vi "PumpValveHeater.vi"() -> ()   [LabVIEW 2015]
uses:
  PumpValve.ctl
  <vilib>/DAQmx/write.llb/DAQmx Write (Digital 1D Bool NChan 1Samp 1Line).vi
  <vilib>/DAQmx/miscellaneous.llb/DAQmx Fill In Error Info.vi
panel:
  in  "On/Off Temp":bool
  in  "Manual Mode Temp":bool
  in  "stop controller":bool
  in  "Set Temp":bool
  in  "Duty cycle % (0-100)":dbl=50.0
  in  "stop PWM":bool
  in  "Steps in a cycle":i32=256
  in  "Cycle time (s)":i32=5
  in  "On/Off (Pump)":bool
  in  "Open/Close (Blue)":bool
  in  "Open/Close (Green)":bool
  in  "Manual Mode Pump/Valve":bool
  out "Invalid fill%":bool
  out "Tank":u32(slide) scale=0.0..100.0
  in  "Drain %":u32
  in  "Fill %":u32
  in  "Drain":bool
  in  "Stop Program":bool
  in  "Fill":bool
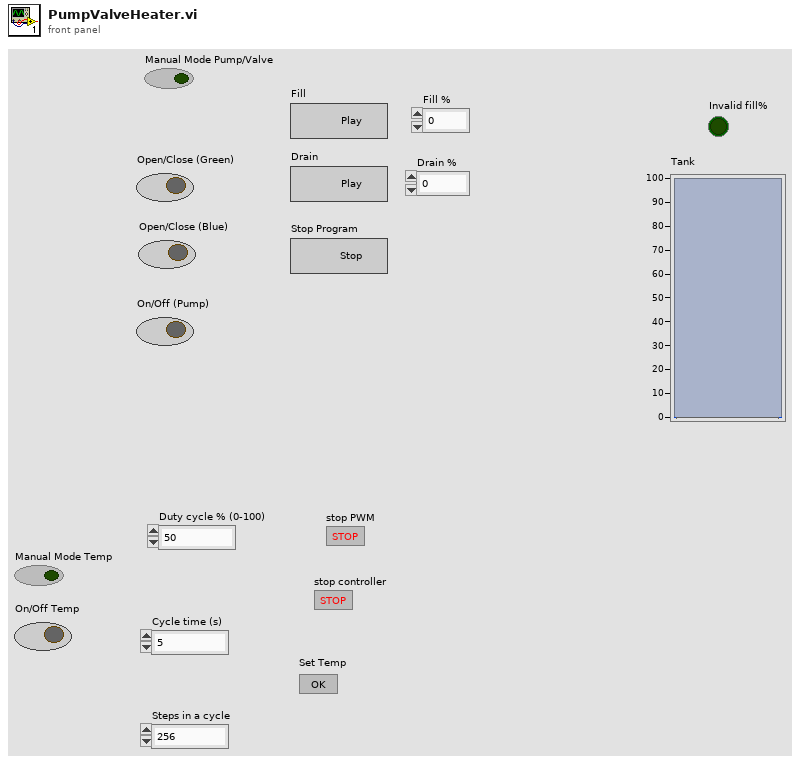
[diagram p1: front panel]
types:
  T1 = typedef "PumpValve.ctl" = enum16{"ManualTemp", "Idle Temp", "Set Temp", "Initialize", "Idle", "Fill", "Drain", "Stop"}
  T2 = cluster{"Open/Close (Green)":bool, "Open/Close (Blue)":bool, "On/Off (Pump)":bool}
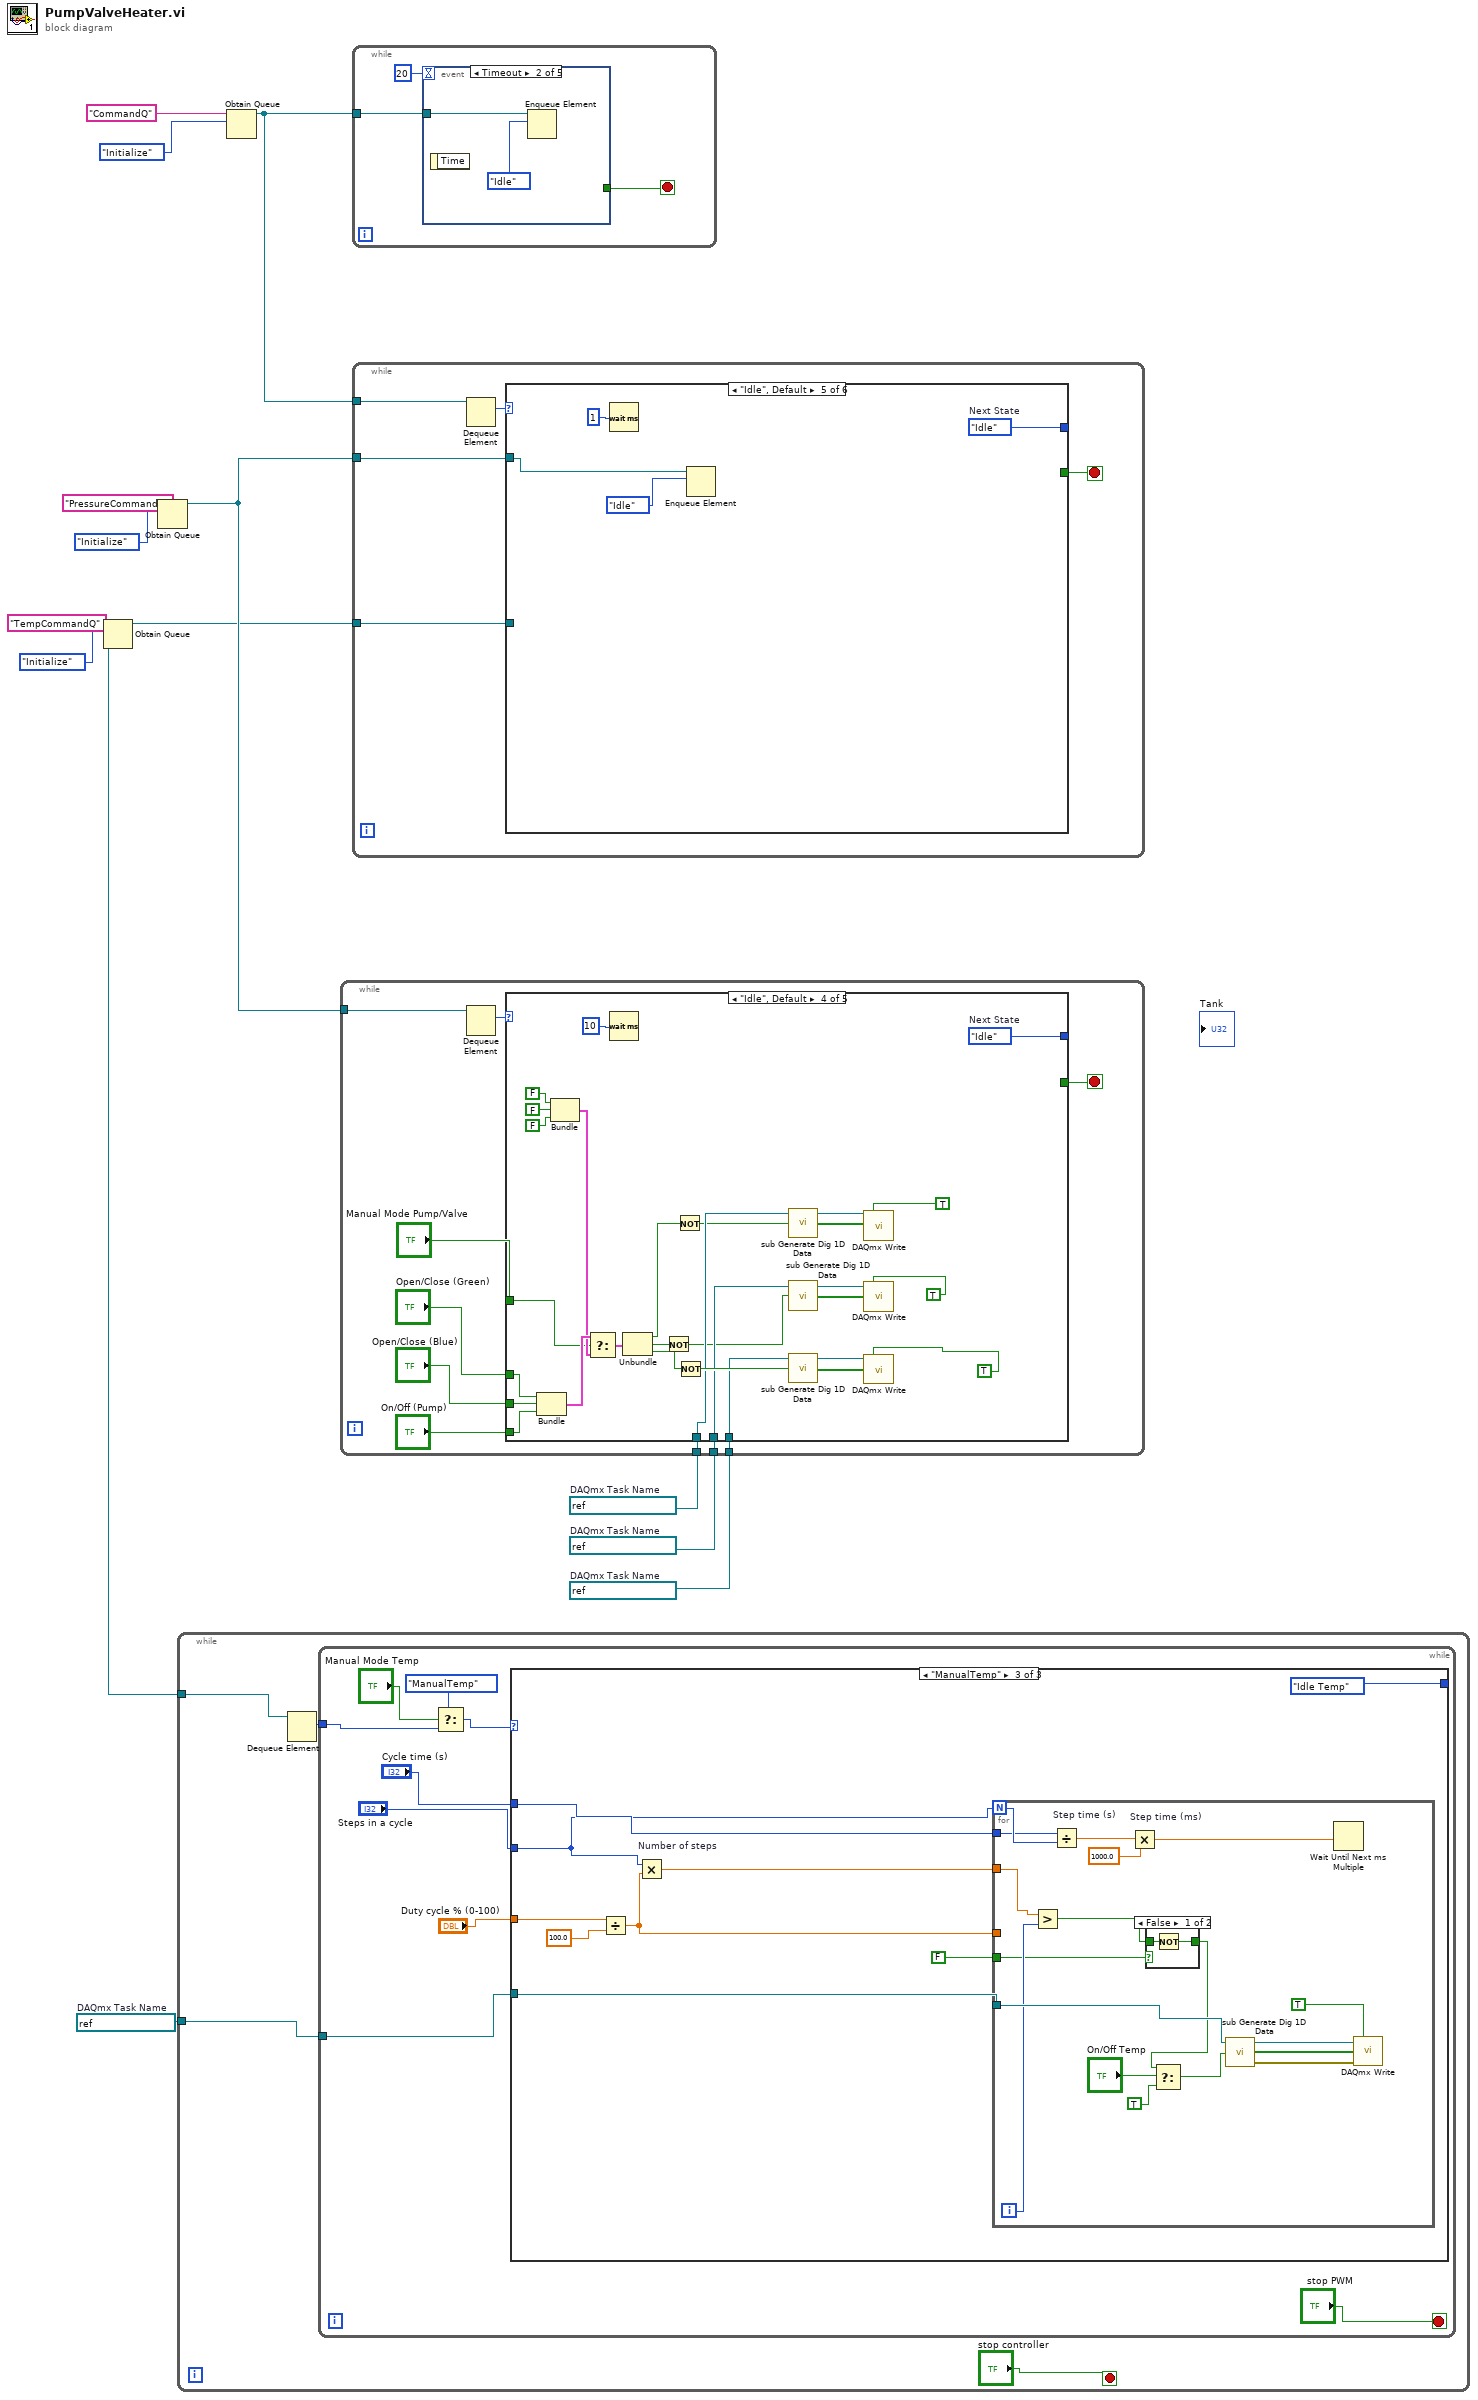
[diagram p0: block diagram]
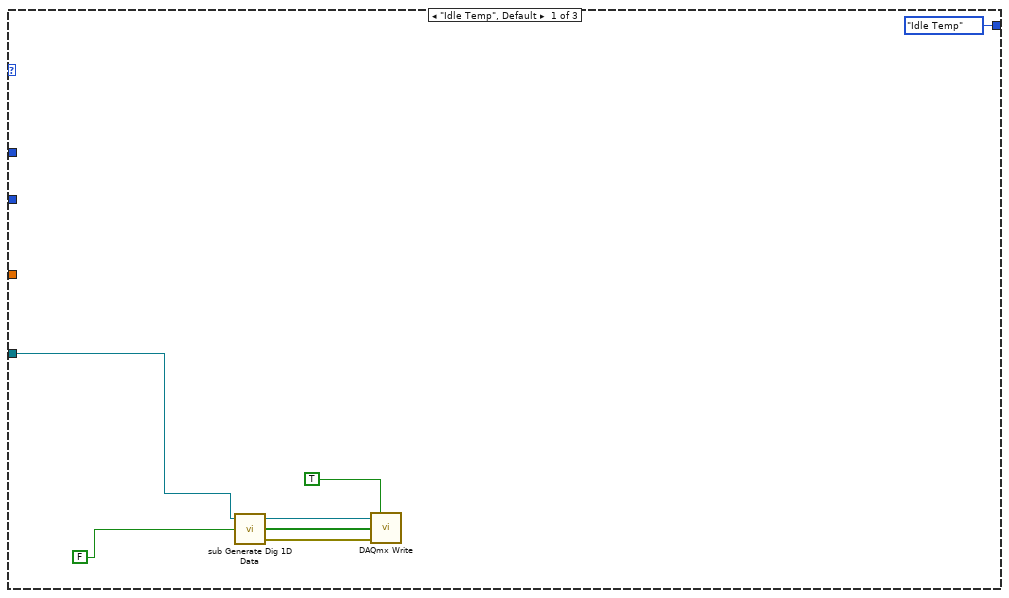
[diagram p2: hidden frame]
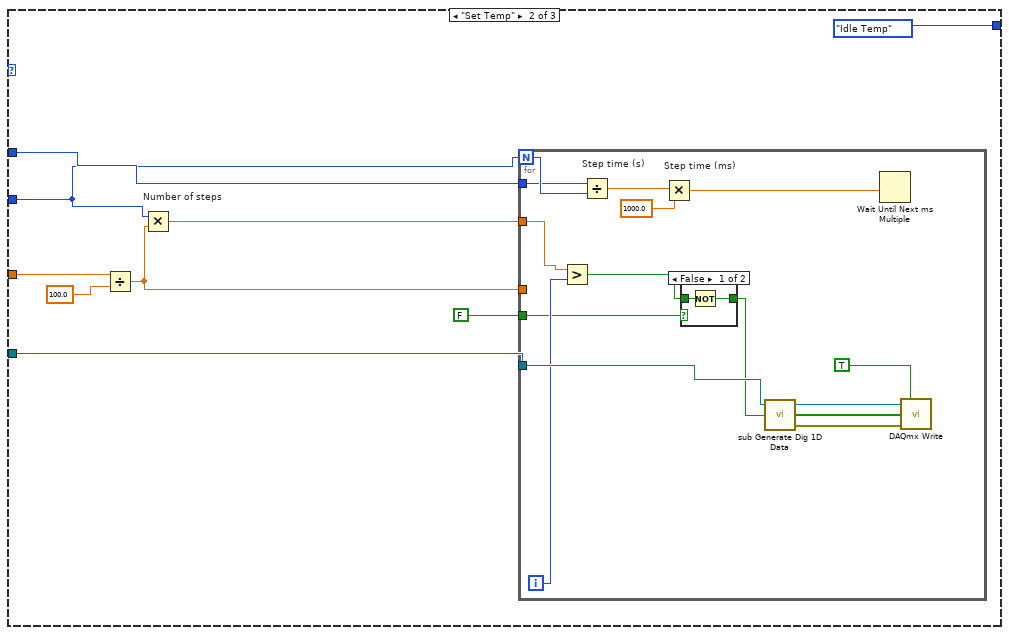
[diagram p3: hidden frame]
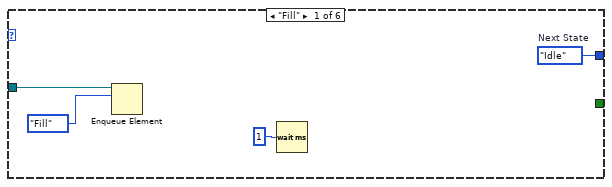
[diagram p6: hidden frame]
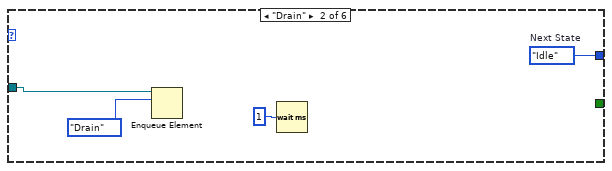
[diagram p7: hidden frame]
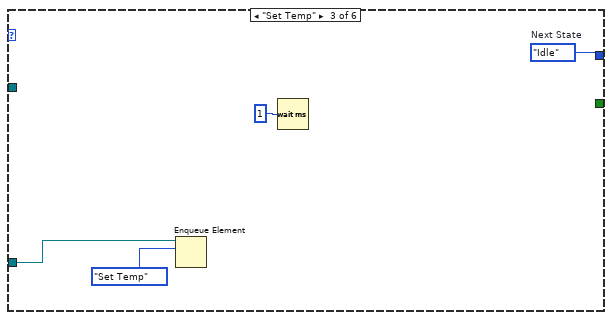
[diagram p8: hidden frame]
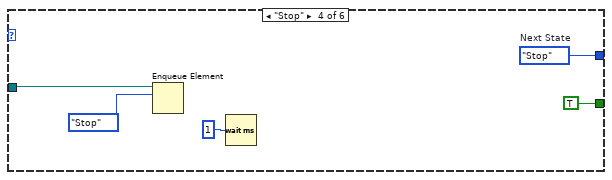
[diagram p9: hidden frame]
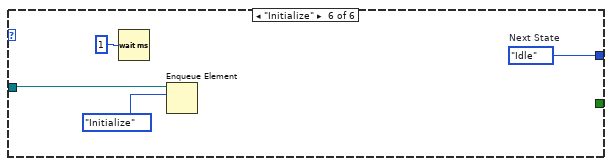
[diagram p10: hidden frame]
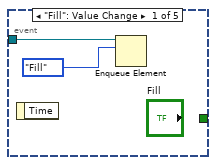
[diagram p11: hidden frame]
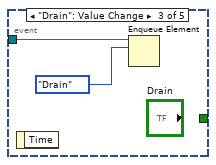
[diagram p12: hidden frame]
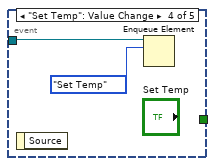
[diagram p13: hidden frame]
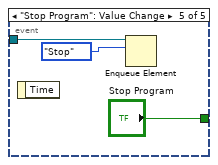
[diagram p14: hidden frame]
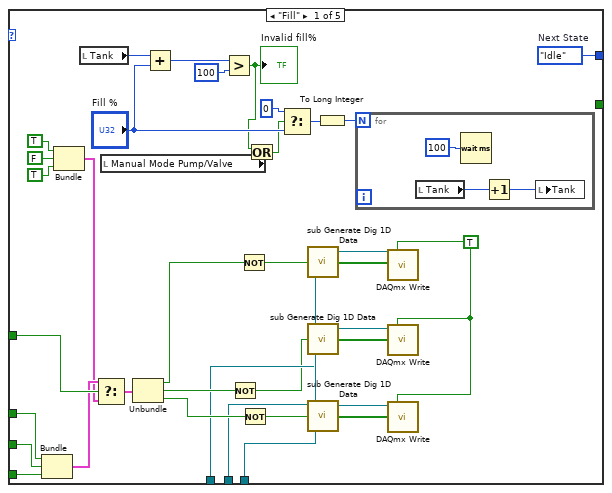
[diagram p15: hidden frame]
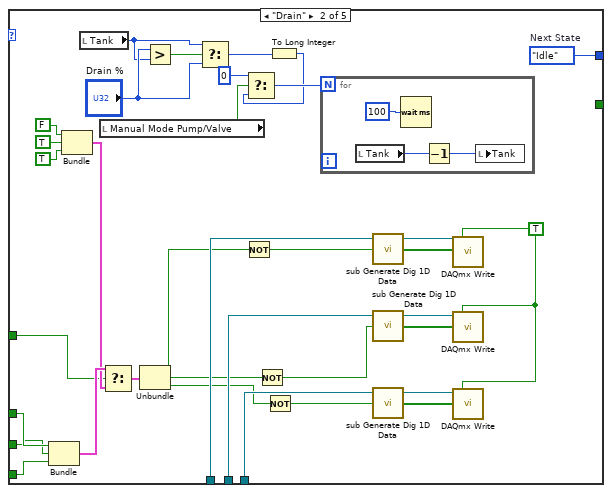
[diagram p16: hidden frame]
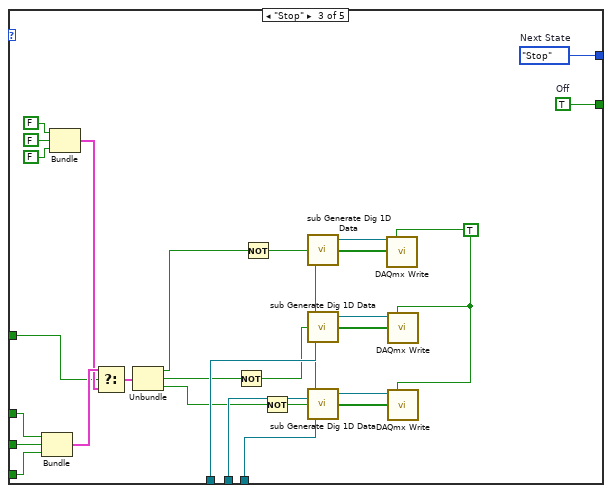
[diagram p17: hidden frame]
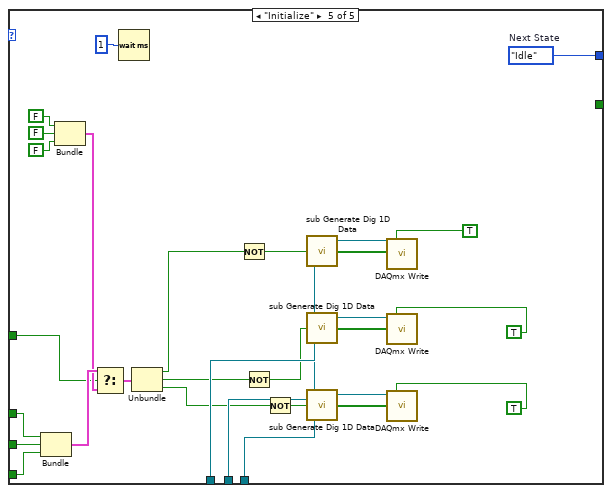
[diagram p18: hidden frame]
diagram:
  w4 = refnum<k21> "DigitalOutBlue"  # DAQmx Task Name
  w9 = refnum<k21> "DigitalOutGreen"  # DAQmx Task Name
  w10 = refnum<k21> "DigitalOutGreen"  # DAQmx Task Name
  w11 = refnum<k21> "DigitalOutGreen"  # DAQmx Task Name
  n1 = Obtain Queue(name (unnamed)="TempCommandQ", element data type=PumpValve."Initialize" ("States")) -> (queue out=w1:refnum<queue>)  [unwired: 3 in, 2 out]
  n2 = Obtain Queue(name (unnamed)="PressureCommandQ", element data type=PumpValve."Initialize" ("States")) -> (queue out=w5:refnum<queue>)  [unwired: 3 in, 2 out]
  n3 = while {
    tunnel: w4 -> [w17]
    tunnel: w1 -> [w16]
    stop <- "stop controller" stop-if-true
    n4 = Dequeue Element(queue=w16) -> (element=w15:T1)  [unwired: 2 in, 3 out]
    n5 = while {
      tunnel: w17 -> [w26]
      tunnel: w15 -> [w21]
      stop <- "stop PWM" stop-if-true
      n6 = Select(t=PumpValve."ManualTemp", s="Manual Mode Temp", f=w21) -> (s? t:f=w20:T1)
      n7 = case shown="\"ManualTemp\"" w20 {
        tunnel: w26 -> [w28 w42 w69]
        tunnel: [PumpValve."Idle Temp" ("States") PumpValve."Idle Temp" ("States") PumpValve."Idle Temp" ("States")] -> _
        tunnel: "Cycle time (s)" -> [_ w36 w63]
        tunnel: "Steps in a cycle" -> [_ w35 w62]
        tunnel: "Duty cycle % (0-100)" -> [_ w34 w61]
        frame "Idle Temp", Default {
          n8 = call <vilib>:"sub Generate Dig 1D Data.vi"("initial value"=FALSE, "task in"=w28) -> ("error out"=w30:errorcluster, "Data"=w31:bool[], "task out"=w32:refnum<k21>)  [unwired: 1 in]
          n9 = call-poly <vilib>:"DAQmx Write.vi"("task/channels in"=w32, "auto start"=TRUE, "data"=w31, "error in"=w30) -> ()  [unwired: 9 in, 3 out]
        }
        frame "Set Temp" {
          n10 = Divide(x=w34, y=100.0) -> (x/y=w40:dbl)
          n11 = Multiply "Number of steps"(x=w35, y=w40) -> (x*y=w39:dbl)
          n12 = for {
            N: w35 -> [w51]
            tunnel: w42 -> [w53]
            tunnel: w40 -> [_]
            tunnel: w36 -> [w50]
            tunnel: w39 -> [w46]
            tunnel: FALSE -> [w43]
            i -> [w45]
            n13 = Greater?(x=w46, y=w45) -> (0:w44:bool)
            n14 = Divide "Step time (s)"(x=w50, y=w51) -> (x/y=w49:dbl)
            n15 = Multiply "Step time (ms)"(x=w49, y=1000.0) -> (x*y=w47:dbl)
            n16 = case shown="False" w43 {
              tunnel: [w58 w60] -> w52
              tunnel: w44 -> [w59 w60]
              frame False {
                n17 = Not(x=w59) -> (.not. x?=w58:bool)
              }
              frame True {
              }
            }
            n18 = call <vilib>:"sub Generate Dig 1D Data.vi"("initial value"=w52, "task in"=w53) -> ("error out"=w56:errorcluster, "Data"=w55:bool[], "task out"=w54:refnum<k21>)  [unwired: 1 in]
            n19 = Wait Until Next ms Multiple(millisecond multiple=w47) -> ()  [unwired: 1 out]
            n20 = call-poly <vilib>:"DAQmx Write.vi"("task/channels in"=w54, "auto start"=TRUE, "data"=w55, "error in"=w56) -> ()  [unwired: 9 in, 3 out]
          }
        }
        frame "ManualTemp" {
          n21 = Divide(x=w61, y=100.0) -> (x/y=w67:dbl)
          n22 = Multiply "Number of steps"(x=w62, y=w67) -> (x*y=w66:dbl)
          n23 = for {
            N: w62 -> [w82]
            tunnel: w69 -> [w83]
            tunnel: w67 -> [_]
            tunnel: w63 -> [w81]
            tunnel: w66 -> [w77]
            tunnel: FALSE -> [w74]
            i -> [w76]
            n24 = Greater?(x=w77, y=w76) -> (0:w75:bool)
            n25 = Divide "Step time (s)"(x=w81, y=w82) -> (x/y=w80:dbl)
            n26 = Multiply "Step time (ms)"(x=w80, y=1000.0) -> (x*y=w78:dbl)
            n27 = case shown="False" w74 {
              tunnel: [w88 w90] -> w72
              tunnel: w75 -> [w89 w90]
              frame False {
                n28 = Not(x=w89) -> (.not. x?=w88:bool)
              }
              frame True {
              }
            }
            n29 = Select(t=w72, s="On/Off Temp", f=TRUE) -> (s? t:f=w71:bool)
            n30 = call <vilib>:"sub Generate Dig 1D Data.vi"("initial value"=w71, "task in"=w83) -> ("error out"=w86:errorcluster, "Data"=w85:bool[], "task out"=w84:refnum<k21>)  [unwired: 1 in]
            n31 = Wait Until Next ms Multiple(millisecond multiple=w78) -> ()  [unwired: 1 out]
            n32 = call-poly <vilib>:"DAQmx Write.vi"("task/channels in"=w84, "auto start"=TRUE, "data"=w85, "error in"=w86) -> ()  [unwired: 9 in, 3 out]
          }
        }
      }
    }
  }
  n33 = Obtain Queue(name (unnamed)="CommandQ", element data type=PumpValve."Initialize" ("States")) -> (queue out=w8:refnum<queue>)  [unwired: 3 in, 2 out]
  n34 = while {
    tunnel: w5 -> [w100]
    tunnel: w11 -> [w91]
    tunnel: w10 -> [w92]
    tunnel: w9 -> [w93]
    stop <- w99 stop-if-true
    n35 = Dequeue Element(queue=w100) -> (element=w98:T1)  [unwired: 2 in, 3 out]
    n36 = case shown="\"Idle\", Default" w98 {
      tunnel: [w137 w175 w206 w236 w266] -> _
      tunnel: [_ _ w179 _ _] -> w99
      tunnel: "Open/Close (Blue)" -> [w123 w151 w187 w219 w246]
      tunnel: "Open/Close (Green)" -> [w122 w152 w188 w220 w247]
      tunnel: "On/Off (Pump)" -> [w121 w150 w186 w218 w245]
      tunnel: "Manual Mode Pump/Valve" -> [w120 w153 w189 w221 w248]
      tunnel: w93 -> [w106 w147 w191 w211 w250]
      tunnel: w92 -> [w105 w148 w192 w210 w251]
      tunnel: w91 -> [w104 w149 w193 w209 w252]
      frame "Fill" {
        w116 = TRUE
        w137 = PumpValve."Idle"  # Next State
        n37 = Bundle("Open/Close (Green)"=w122, "Open/Close (Blue)"=w123, "On/Off (Pump)"=w121) -> (w119:T2)  [unwired: 1 in]
        n38 = Bundle(TRUE, FALSE, TRUE) -> (w118:cluster{bool, bool, bool})  [unwired: 1 in]
        n39 = local read "Tank"() -> (w136:u32)
        n40 = Select(t=w119, s=w120, f=w118) -> (s? t:f=w117:T2)
        n41 = local read "Manual Mode Pump/Valve"() -> (w125:bool)
        n42 = Unbundle(w117) -> ("Open/Close (Green)"=w109:bool, "Open/Close (Blue)"=w108:bool, "On/Off (Pump)"=w107:bool)
        n43 = Add(x=w136, y="Fill %") -> (x+y=w134:u32)
        n44 = Greater?(x=w134, y=u32 100) -> (0:w126:bool)
        "Invalid fill%" <- w126
        n45 = Not(x=w108) -> (.not. x?=w101:bool)
        n46 = Not(x=w109) -> (.not. x?=w102:bool)
        n47 = Not(x=w107) -> (.not. x?=w103:bool)
        n48 = Or(x=w126, y=w125) -> (x .or. y?=w124:bool)
        n49 = Select(t=u32 0, s=w124, f="Fill %") -> (s? t:f=w131:u32)
        n50 = call <vilib>:"sub Generate Dig 1D Data.vi"("initial value"=w102, "task in"=w104) -> ("Data"=w111:bool[], "task out"=w115:refnum<k21>)  [unwired: 1 in, 1 out]
        n51 = call <vilib>:"sub Generate Dig 1D Data.vi"("initial value"=w101, "task in"=w105) -> ("Data"=w112:bool[], "task out"=w114:refnum<k21>)  [unwired: 1 in, 1 out]
        n52 = call <vilib>:"sub Generate Dig 1D Data.vi"("initial value"=w103, "task in"=w106) -> ("Data"=w110:bool[], "task out"=w113:refnum<k21>)  [unwired: 1 in, 1 out]
        n53 = To Long Integer(number=w131) -> (32bit integer=w130:i32)
        n54 = for {
          N: w130 -> [_]
          n55 = local read "Tank"() -> (w140:u32)
          n56 = Wait (ms)(milliseconds to wait=u32 100 ("y")) -> ()  [unwired: 1 out]
          n57 = Increment(x=w140) -> (x+1=w139:u32)
          n58 = local write "Tank"(w139) -> ()
        }
        n59 = call-poly <vilib>:"DAQmx Write.vi"("task/channels in"=w115, "auto start"=w116, "data"=w111) -> ()  [unwired: 10 in, 3 out]
        n60 = call-poly <vilib>:"DAQmx Write.vi"("task/channels in"=w114, "auto start"=w116, "data"=w112) -> ()  [unwired: 10 in, 3 out]
        n61 = call-poly <vilib>:"DAQmx Write.vi"("task/channels in"=w113, "auto start"=w116, "data"=w110) -> ()  [unwired: 10 in, 3 out]
      }
      frame "Drain" {
        w157 = TRUE
        w175 = PumpValve."Idle"  # Next State
        n62 = Bundle("Open/Close (Green)"=w152, "Open/Close (Blue)"=w151, "On/Off (Pump)"=w150) -> (w155:T2)  [unwired: 1 in]
        n63 = Bundle(FALSE, TRUE, TRUE) -> (w154:cluster{bool, bool, bool})  [unwired: 1 in]
        n64 = local read "Tank"() -> (w172:u32)
        n65 = local read "Manual Mode Pump/Valve"() -> (w167:bool)
        n66 = Select(t=w155, s=w153, f=w154) -> (s? t:f=w156:T2)
        n67 = Unbundle(w156) -> ("Open/Close (Green)"=w146:bool, "Open/Close (Blue)"=w145:bool, "On/Off (Pump)"=w144:bool)
        n68 = Greater?(x="Drain %", y=w172) -> (0:w168:bool)
        n69 = Select(t=w172, s=w168, f="Drain %") -> (s? t:f=w174:u32)
        n70 = Not(x=w146) -> (.not. x?=w142:bool)
        n71 = Not(x=w145) -> (.not. x?=w141:bool)
        n72 = Not(x=w144) -> (.not. x?=w143:bool)
        n73 = To Long Integer(number=w174) -> (32bit integer=w164:i32)
        n74 = Select(t=0, s=w167, f=w164) -> (s? t:f=w165:i32)
        n75 = for {
          N: w165 -> [_]
          n76 = local read "Tank"() -> (w177:u32)
          n77 = Wait (ms)(milliseconds to wait=u32 100) -> ()  [unwired: 1 out]
          n78 = Decrement(x=w177) -> (x-1=w178:u32)
          n79 = local write "Tank"(w178) -> ()
        }
        n80 = call <vilib>:"sub Generate Dig 1D Data.vi"("initial value"=w142, "task in"=w149) -> ("Data"=w162:bool[], "task out"=w158:refnum<k21>)  [unwired: 1 in, 1 out]
        n81 = call <vilib>:"sub Generate Dig 1D Data.vi"("initial value"=w141, "task in"=w148) -> ("Data"=w161:bool[], "task out"=w159:refnum<k21>)  [unwired: 1 in, 1 out]
        n82 = call <vilib>:"sub Generate Dig 1D Data.vi"("initial value"=w143, "task in"=w147) -> ("Data"=w163:bool[], "task out"=w160:refnum<k21>)  [unwired: 1 in, 1 out]
        n83 = call-poly <vilib>:"DAQmx Write.vi"("task/channels in"=w158, "auto start"=w157, "data"=w162) -> ()  [unwired: 10 in, 3 out]
        n84 = call-poly <vilib>:"DAQmx Write.vi"("task/channels in"=w159, "auto start"=w157, "data"=w161) -> ()  [unwired: 10 in, 3 out]
        n85 = call-poly <vilib>:"DAQmx Write.vi"("task/channels in"=w160, "auto start"=w157, "data"=w163) -> ()  [unwired: 10 in, 3 out]
      }
      frame "Stop" {
        w200 = TRUE
        w179 = TRUE  # Off
        w206 = PumpValve."Stop"  # Next State
        n86 = Bundle("Open/Close (Green)"=w188, "Open/Close (Blue)"=w187, "On/Off (Pump)"=w186) -> (w202:T2)  [unwired: 1 in]
        n87 = Bundle(FALSE, FALSE, FALSE) -> (w190:cluster{bool, bool, bool})  [unwired: 1 in]
        n88 = Select(t=w202, s=w189, f=w190) -> (s? t:f=w201:T2)
        n89 = Unbundle(w201) -> ("Open/Close (Green)"=w185:bool, "Open/Close (Blue)"=w184:bool, "On/Off (Pump)"=w183:bool)
        n90 = Not(x=w184) -> (.not. x?=w180:bool)
        n91 = Not(x=w185) -> (.not. x?=w181:bool)
        n92 = Not(x=w183) -> (.not. x?=w182:bool)
        n93 = call <vilib>:"sub Generate Dig 1D Data.vi"("initial value"=w181, "task in"=w193) -> ("Data"=w195:bool[], "task out"=w199:refnum<k21>)  [unwired: 1 in, 1 out]
        n94 = call <vilib>:"sub Generate Dig 1D Data.vi"("initial value"=w180, "task in"=w192) -> ("Data"=w196:bool[], "task out"=w198:refnum<k21>)  [unwired: 1 in, 1 out]
        n95 = call <vilib>:"sub Generate Dig 1D Data.vi"("initial value"=w182, "task in"=w191) -> ("Data"=w194:bool[], "task out"=w197:refnum<k21>)  [unwired: 1 in, 1 out]
        n96 = call-poly <vilib>:"DAQmx Write.vi"("task/channels in"=w199, "auto start"=w200, "data"=w195) -> ()  [unwired: 10 in, 3 out]
        n97 = call-poly <vilib>:"DAQmx Write.vi"("task/channels in"=w198, "auto start"=w200, "data"=w196) -> ()  [unwired: 10 in, 3 out]
        n98 = call-poly <vilib>:"DAQmx Write.vi"("task/channels in"=w197, "auto start"=w200, "data"=w194) -> ()  [unwired: 10 in, 3 out]
      }
      frame "Idle", Default {
        w236 = PumpValve."Idle"  # Next State
        n99 = Bundle("Open/Close (Green)"=w220, "Open/Close (Blue)"=w219, "On/Off (Pump)"=w218) -> (w231:T2)  [unwired: 1 in]
        n100 = Bundle(FALSE, FALSE, FALSE) -> (w222:cluster{bool, bool, bool})  [unwired: 1 in]
        n101 = Select(t=w231, s=w221, f=w222) -> (s? t:f=w230:T2)
        n102 = Wait (ms)(milliseconds to wait=u32 10) -> ()  [unwired: 1 out]
        n103 = Unbundle(w230) -> ("Open/Close (Green)"=w217:bool, "Open/Close (Blue)"=w216:bool, "On/Off (Pump)"=w215:bool)
        n104 = Not(x=w216) -> (.not. x?=w207:bool)
        n105 = Not(x=w217) -> (.not. x?=w208:bool)
        n106 = Not(x=w215) -> (.not. x?=w214:bool)
        n107 = call <vilib>:"sub Generate Dig 1D Data.vi"("initial value"=w208, "task in"=w209) -> ("Data"=w224:bool[], "task out"=w228:refnum<k21>)  [unwired: 1 in, 1 out]
        n108 = call <vilib>:"sub Generate Dig 1D Data.vi"("initial value"=w207, "task in"=w210) -> ("Data"=w225:bool[], "task out"=w227:refnum<k21>)  [unwired: 1 in, 1 out]
        n109 = call <vilib>:"sub Generate Dig 1D Data.vi"("initial value"=w214, "task in"=w211) -> ("Data"=w223:bool[], "task out"=w226:refnum<k21>)  [unwired: 1 in, 1 out]
        n110 = call-poly <vilib>:"DAQmx Write.vi"("task/channels in"=w228, "auto start"=TRUE, "data"=w224) -> ()  [unwired: 10 in, 3 out]
        n111 = call-poly <vilib>:"DAQmx Write.vi"("task/channels in"=w227, "auto start"=TRUE, "data"=w225) -> ()  [unwired: 10 in, 3 out]
        n112 = call-poly <vilib>:"DAQmx Write.vi"("task/channels in"=w226, "auto start"=TRUE, "data"=w223) -> ()  [unwired: 10 in, 3 out]
      }
      frame "Initialize" {
        w266 = PumpValve."Idle"  # Next State
        n113 = Bundle("Open/Close (Green)"=w247, "Open/Close (Blue)"=w246, "On/Off (Pump)"=w245) -> (w261:T2)  [unwired: 1 in]
        n114 = Bundle(FALSE, FALSE, FALSE) -> (w249:cluster{bool, bool, bool})  [unwired: 1 in]
        n115 = Select(t=w261, s=w248, f=w249) -> (s? t:f=w260:T2)
        n116 = Wait (ms)(milliseconds to wait=u32 1) -> ()  [unwired: 1 out]
        n117 = Unbundle(w260) -> ("Open/Close (Green)"=w244:bool, "Open/Close (Blue)"=w243:bool, "On/Off (Pump)"=w242:bool)
        n118 = Not(x=w244) -> (.not. x?=w238:bool)
        n119 = Not(x=w243) -> (.not. x?=w237:bool)
        n120 = Not(x=w242) -> (.not. x?=w241:bool)
        n121 = call <vilib>:"sub Generate Dig 1D Data.vi"("initial value"=w238, "task in"=w252) -> ("Data"=w254:bool[], "task out"=w258:refnum<k21>)  [unwired: 1 in, 1 out]
        n122 = call <vilib>:"sub Generate Dig 1D Data.vi"("initial value"=w237, "task in"=w251) -> ("Data"=w255:bool[], "task out"=w257:refnum<k21>)  [unwired: 1 in, 1 out]
        n123 = call <vilib>:"sub Generate Dig 1D Data.vi"("initial value"=w241, "task in"=w250) -> ("Data"=w253:bool[], "task out"=w256:refnum<k21>)  [unwired: 1 in, 1 out]
        n124 = call-poly <vilib>:"DAQmx Write.vi"("task/channels in"=w258, "auto start"=TRUE, "data"=w254) -> ()  [unwired: 10 in, 3 out]
        n125 = call-poly <vilib>:"DAQmx Write.vi"("task/channels in"=w257, "auto start"=TRUE, "data"=w255) -> ()  [unwired: 10 in, 3 out]
        n126 = call-poly <vilib>:"DAQmx Write.vi"("task/channels in"=w256, "auto start"=TRUE, "data"=w253) -> ()  [unwired: 10 in, 3 out]
      }
    }
  }
  n127 = while {
    tunnel: w8 -> [w268]
    stop <- w267 stop-if-true
    n128 = event shown="[1] Timeout" {
      selector: _ -> [_ _ _ _ _]
      dyn-events: _ -> [_ _ _ _ _]
      timeout: 20 -> [_ _ _ _ _]
      tunnel: w268 -> [w271 w273 w275 w276 w280]
      tunnel: [_ _ _ _ "Stop Program"] -> w267
      event "Fill": Value Change {
        n129 = event-data() -> ()  [unwired: 1 in, 1 out]
        n130 = Enqueue Element(queue=w271, element=PumpValve."Fill" ("States")) -> ()  [unwired: 2 in, 3 out]
      }
      event Timeout {
        n131 = event-data() -> ()  [unwired: 1 in, 1 out]
        n132 = Enqueue Element(queue=w273, element=PumpValve."Idle" ("States")) -> ()  [unwired: 2 in, 3 out]
      }
      event "Drain": Value Change {
        n133 = event-data() -> ()  [unwired: 1 in, 1 out]
        n134 = Enqueue Element(queue=w275, element=PumpValve."Drain" ("States")) -> ()  [unwired: 2 in, 3 out]
      }
      event "Set Temp": Value Change {
        n135 = event-data() -> ()  [unwired: 1 in, 1 out]
        n136 = Enqueue Element(queue=w276, element=PumpValve."Set Temp" ("States")) -> ()  [unwired: 2 in, 3 out]
      }
      event "Stop Program": Value Change {
        n137 = event-data() -> ()  [unwired: 1 in, 1 out]
        n138 = Enqueue Element(queue=w280, element=PumpValve."Stop" ("States")) -> ()  [unwired: 2 in, 3 out]
      }
    }
  }
  n139 = while {
    tunnel: w8 -> [w284]
    tunnel: w5 -> [w283]
    tunnel: w1 -> [w281]
    stop <- w282 stop-if-true
    n140 = Dequeue Element(queue=w284) -> (element=w285:T1)  [unwired: 2 in, 3 out]
    n141 = case shown="\"Idle\", Default" w285 {
      tunnel: [w289 w293 w295 w302 w306 w310] -> _
      tunnel: w283 -> [w286 w290 _ w299 w303 w307]
      tunnel: [_ _ _ TRUE _ _] -> w282
      tunnel: w281 -> [_ _ w294 _ _ _]
      frame "Fill" {
        w289 = PumpValve."Idle"  # Next State
        n142 = Enqueue Element(queue=w286, element=PumpValve."Fill" ("States")) -> ()  [unwired: 2 in, 3 out]
        n143 = Wait (ms)(milliseconds to wait=u32 1) -> ()  [unwired: 1 out]
      }
      frame "Drain" {
        w293 = PumpValve."Idle"  # Next State
        n144 = Enqueue Element(queue=w290, element=PumpValve."Drain" ("States")) -> ()  [unwired: 2 in, 3 out]
        n145 = Wait (ms)(milliseconds to wait=u32 1) -> ()  [unwired: 1 out]
      }
      frame "Set Temp" {
        w295 = PumpValve."Idle"  # Next State
        n146 = Enqueue Element(queue=w294, element=PumpValve."Set Temp" ("States")) -> ()  [unwired: 2 in, 3 out]
        n147 = Wait (ms)(milliseconds to wait=u32 1) -> ()  [unwired: 1 out]
      }
      frame "Stop" {
        w302 = PumpValve."Stop"  # Next State
        n148 = Enqueue Element(queue=w299, element=PumpValve."Stop" ("States")) -> ()  [unwired: 2 in, 3 out]
        n149 = Wait (ms)(milliseconds to wait=u32 1) -> ()  [unwired: 1 out]
      }
      frame "Idle", Default {
        w306 = PumpValve."Idle"  # Next State
        n150 = Wait (ms)(milliseconds to wait=u32 1) -> ()  [unwired: 1 out]
        n151 = Enqueue Element(queue=w303, element=PumpValve."Idle" ("States")) -> ()  [unwired: 2 in, 3 out]
      }
      frame "Initialize" {
        w310 = PumpValve."Idle"  # Next State
        n152 = Wait (ms)(milliseconds to wait=u32 1) -> ()  [unwired: 1 out]
        n153 = Enqueue Element(queue=w307, element=PumpValve."Initialize" ("States")) -> ()  [unwired: 2 in, 3 out]
      }
    }
  }
